vi "test_CCDSetAndGetTimerResolution.vi"(7 "Test should pass":bool=TRUE, 8 "error in":errorcluster, 9 "tear down connection":bool=TRUE, 10 "set-up a connection":bool=TRUE, 11 "device selection":enum16{"monochromator", "CCD", "SCD"}(ring)=enum."CCD") -> (0 "error out":errorcluster)   [LabVIEW 2023]
uses:
  <vilib>/addons/_JKI Toolkits/Caraya/classes/Test/Test.lvclass
  <vilib>/addons/_JKI Toolkits/Caraya/classes/Assert/Assert.lvclass
  <vilib>/addons/_JKI Toolkits/Caraya/classes/Assert/Assert Equal Value and Type_Variant.vi
  Classes/CCD/GainTokenEnum.ctl
  Classes/CCD/CCD.lvclass
  <vilib>/addons/_JKI Toolkits/Caraya/classes/Assert/Assert Not Error.vi
  Classes/CCD/TimerResolutionEnum.ctl
panel:
  # "Connector Pane"
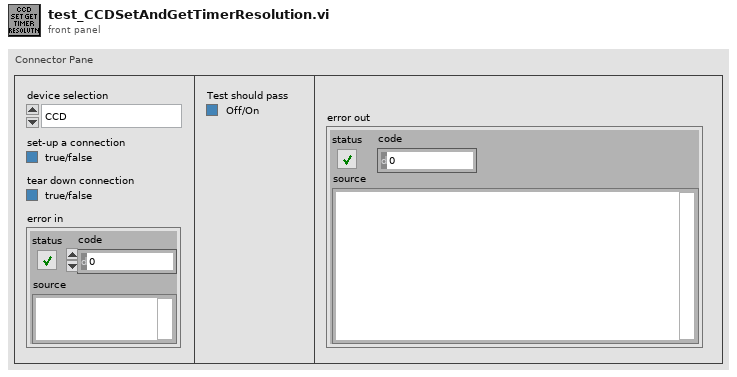
[diagram p1: front panel]
types:
  T1 = typedef "CCD.lvclass/TimerResolutionEnum.ctl" = enum16{"0 - Sets the timer resolution to 1000 microseconds", "1 - Sets the timer resolution to 1 microsecond"}
  T2 = typedef "CCD.lvclass/GainTokenEnum.ctl" = enum16{"High Light", "Best Dynamic Range", "High Sensitivity"}
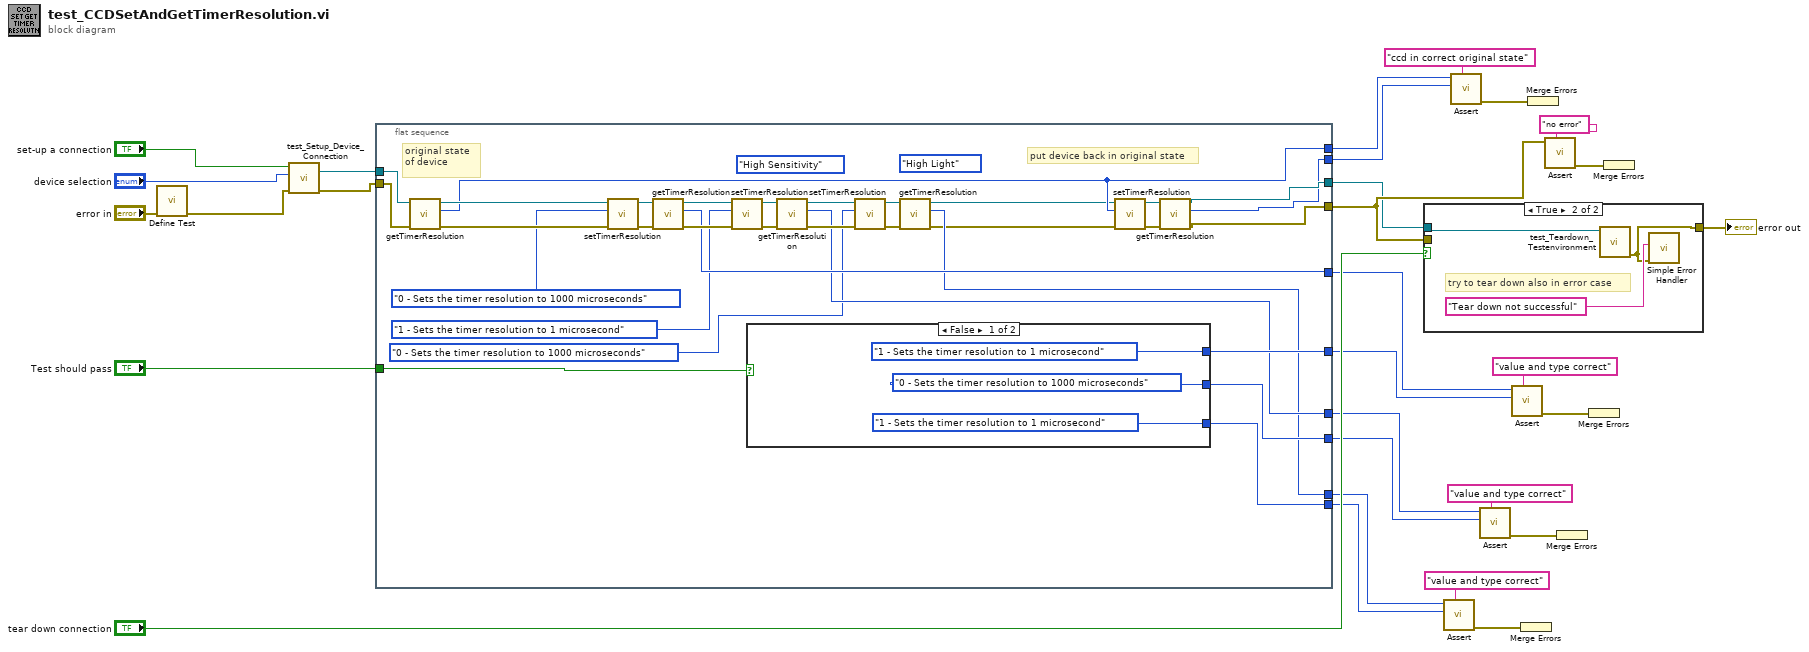
[diagram p0: block diagram]
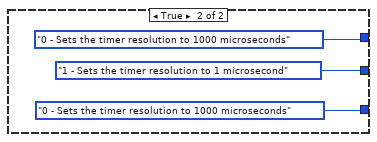
[diagram p2: hidden frame]
diagram:
  n1 = call <vilib>:"Define Test.vi"("error in (no error)"="error in") -> ("error out"=w4:errorcluster)  [unwired: 9 in, 1 out]
  n2 = call "test_Setup_Device_Connection.vi"("error in (no error)"=w4, "device selection"="device selection", "set-up a connection"="set-up a connection") -> ("error out"=w5:errorcluster, "CCD out"=w3:refnum<class "CCD.lvclass">)  [unwired: 5 in, 2 out]
  n3 = flat-sequence {
    tunnel: w5 -> [w59]
    tunnel: w3 -> [w60]
    tunnel: [w43] -> w24
    tunnel: "Test should pass" -> [w61]
    tunnel: [w42] -> w23
    tunnel: [w41] -> w20
    tunnel: [w44] -> w19
    tunnel: [w40] -> w18
    tunnel: [w38] -> w16
    tunnel: [w35] -> w14
    tunnel: [w39] -> w17
    tunnel: [w37] -> w15
    tunnel: [w36] -> w13
    frame #0 {
      (unwired) GainTokenEnum."High Light" ("gain token (enum)")
      (unwired) GainTokenEnum."High Sensitivity" ("gain token (enum)")
      # "put device back in original state"
      # "original state of device"
      n4 = call "getTimerResolution.vi"("error in (no error)"=w59, "CCD in"=w60) -> ("error out"=w45:errorcluster, "resolution"=w44:T1, "CCD out"=w46:refnum<class "CCD.lvclass">)  [unwired: 6 in, 1 out]
      n5 = call "setTimerResolution.vi"("error in (no error)"=w45, "resolution"=TimerResolutionEnum."0 - Sets the timer resolution to 1000 microseconds", "CCD in"=w46) -> ("error out"=w50:errorcluster, "CCD out"=w49:refnum<class "CCD.lvclass">)  [unwired: 5 in, 2 out]
      n6 = call "getTimerResolution.vi"("error in (no error)"=w50, "CCD in"=w49) -> ("error out"=w54:errorcluster, "resolution"=w40:T1, "CCD out"=w53:refnum<class "CCD.lvclass">)  [unwired: 6 in, 1 out]
      n7 = call "setTimerResolution.vi"("error in (no error)"=w54, "resolution"=TimerResolutionEnum."1 - Sets the timer resolution to 1 microsecond", "CCD in"=w53) -> ("error out"=w51:errorcluster, "CCD out"=w52:refnum<class "CCD.lvclass">)  [unwired: 5 in, 2 out]
      n8 = case shown="False" w61 {
        tunnel: [TimerResolutionEnum."1 - Sets the timer resolution to 1 microsecond" ("resolution") TimerResolutionEnum."0 - Sets the timer resolution to 1000 microseconds" ("resolution")] -> w39
        tunnel: [TimerResolutionEnum."0 - Sets the timer resolution to 1000 microseconds" ("resolution") TimerResolutionEnum."1 - Sets the timer resolution to 1 microsecond" ("resolution")] -> w37
        tunnel: [TimerResolutionEnum."1 - Sets the timer resolution to 1 microsecond" ("resolution") TimerResolutionEnum."0 - Sets the timer resolution to 1000 microseconds" ("resolution")] -> w36
        frame False {
        }
        frame True {
        }
      }
      n9 = call "getTimerResolution.vi"("error in (no error)"=w51, "CCD in"=w52) -> ("error out"=w56:errorcluster, "resolution"=w38:T1, "CCD out"=w55:refnum<class "CCD.lvclass">)  [unwired: 6 in, 1 out]
      n10 = call "setTimerResolution.vi"("error in (no error)"=w56, "resolution"=TimerResolutionEnum."0 - Sets the timer resolution to 1000 microseconds", "CCD in"=w55) -> ("error out"=w48:errorcluster, "CCD out"=w47:refnum<class "CCD.lvclass">)  [unwired: 5 in, 2 out]
      n11 = call "getTimerResolution.vi"("error in (no error)"=w48, "CCD in"=w47) -> ("error out"=w30:errorcluster, "resolution"=w35:T1, "CCD out"=w31:refnum<class "CCD.lvclass">)  [unwired: 6 in, 1 out]
      n12 = call "setTimerResolution.vi"("error in (no error)"=w30, "resolution"=w44, "CCD in"=w31) -> ("error out"=w57:errorcluster, "CCD out"=w58:refnum<class "CCD.lvclass">)  [unwired: 5 in, 2 out]
      n13 = call "getTimerResolution.vi"("error in (no error)"=w57, "CCD in"=w58) -> ("error out"=w43:errorcluster, "resolution"=w41:T1, "CCD out"=w42:refnum<class "CCD.lvclass">)  [unwired: 6 in, 1 out]
    }
  }
  n14 = case shown="True" "tear down connection" {
    tunnel: w23 -> [_ w70]
    tunnel: [w68 w69] -> w6
    tunnel: w24 -> [w68 _]
    frame False {
    }
    frame True {
      # "try to tear down also in error case"
      n15 = call "test_Teardown_Testenvironment.vi"("GenericDevice.lvclass"=w70) -> ("error out"=w69:errorcluster)  [unwired: 9 in, 1 out]
      n16 = call <vilib>:"Simple Error Handler.vi"("error source (\" \")"="Tear down not successful" ("error source (\" \")"), "error in (no error)"=w69) -> ()  [unwired: 3 in, 5 out]
    }
  }
  "error out" <- w6
  n17 = call-poly <vilib>:"Assert.vi"("Label"="value and type correct" ("Label (VI Title)"), "Y"=w13, "X"=w14) -> ("error out"=w12:errorcluster)  [unwired: 7 in, 1 out]
  n18 = call-poly <vilib>:"Assert.vi"("Label"="ccd in correct original state" ("Label (VI Title)"), "Y"=w20, "X"=w19) -> ("error out"=w22:errorcluster)  [unwired: 7 in, 1 out]
  n19 = call-poly <vilib>:"Assert.vi"("Label"="value and type correct" ("Label (VI Title)"), "Y"=w15, "X"=w16) -> ("error out"=w8:errorcluster)  [unwired: 7 in, 1 out]
  n20 = call-poly <vilib>:"Assert.vi"("Label"="value and type correct" ("Label (VI Title)"), "Y"=w17, "X"=w18) -> ("error out"=w9:errorcluster)  [unwired: 7 in, 1 out]
  n21 = Merge Errors(w12) -> ()  [unwired: 1 out]
  n22 = Merge Errors(w22) -> ()  [unwired: 1 out]
  n23 = call-poly <vilib>:"Assert.vi"("Label"="no error" ("Label (VI Title)"), "Not Error?"=w24) -> ("error out"=w26:errorcluster)  [unwired: 8 in, 1 out]
  n24 = Merge Errors(w8) -> ()  [unwired: 1 out]
  n25 = Merge Errors(w9) -> ()  [unwired: 1 out]
  n26 = Merge Errors(w26) -> ()  [unwired: 1 out]
